vi "StepperDecision.vi"(4 "Last Pos":dbl, 5 "Steplength(ms)":dbl, 6 "Waittime":u32, 7 "StepMode":enum16{"Use Timing", "Use Encoder"}(ring), 8 "act Pos":dbl, 9 "millisecond timer value":u32, 10 "Moving":bool) -> (0 "f":i32, 3 "millisecond timer value 2":u32)   [LabVIEW 2011]
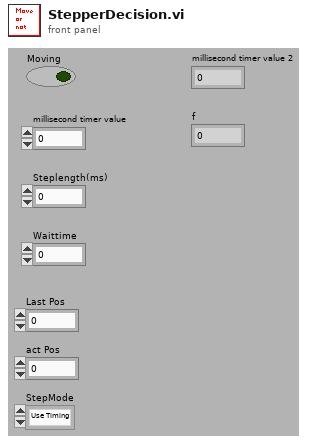
[diagram p1: front panel]
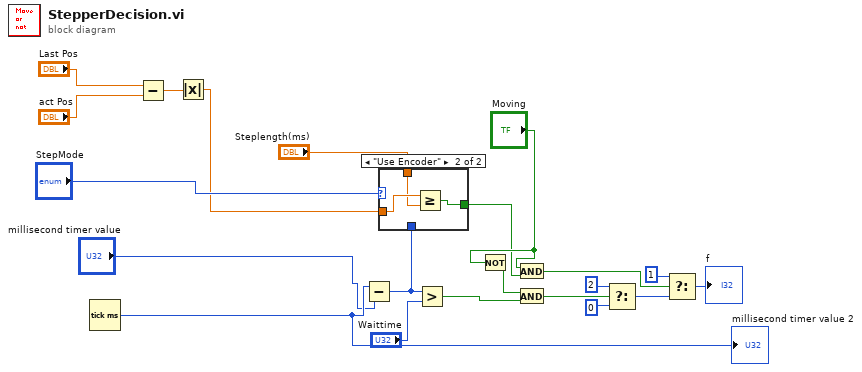
[diagram p0: block diagram]
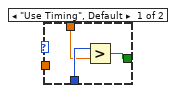
[diagram p2: hidden frame]
diagram:
  n1 = Tick Count (ms)() -> (millisecond timer value=w8:u32)
  "millisecond timer value 2" <- w8
  n2 = Subtract(x="Last Pos", y="act Pos") -> (x-y=w2:dbl)
  n3 = Absolute Value(x=w2) -> (abs(x)=w1:dbl)
  n4 = Subtract(x=w8, y="millisecond timer value") -> (x-y=w14:u32)
  n5 = case shown="\"Use Encoder\"" "StepMode" {
    tunnel: w14 -> [w24 _]
    tunnel: [w23 w27] -> w11
    tunnel: "Steplength(ms)" -> [w22 w25]
    tunnel: w1 -> [_ w26]
    frame "Use Timing", Default {
      n6 = Greater?(x=w24, y=w22) -> (0:w23:bool)
    }
    frame "Use Encoder" {
      n7 = Greater Or Equal?(x=w26, y=w25) -> (x >= y?=w27:bool)
    }
  }
  n8 = Greater?(x=w14, y="Waittime") -> (0:w6:bool)
  n9 = Not(x="Moving") -> (.not. x?=w13:bool)
  n10 = And(x="Moving", y=w11) -> (x .and. y?=w16:bool)
  n11 = And(x=w13, y=w6) -> (x .and. y?=w9:bool)
  n12 = Select(t=2, s=w9, f=0) -> (s? t:f=w20:i32)
  n13 = Select(t=1, s=w16, f=w20) -> (s? t:f=→"f":i32)
